vi "SYST_COMM_GPIB_RDEV_OPEN.vi"(0 "VISA IN":refnum<visa-resource-name>, 1 "Address":i32, 2 "Timeout":i32, 5 "error in":errorcluster, 7 "Bus":i32) -> (14 "VISA Out":refnum<visa-resource-name>, 19 "error out":errorcluster)   [LabVIEW 2018, in "PNA-X.lvlib"]
doc: "SYSTem:COMMunicate:GPIB:RDEVice:OPEN <bus>, <addr>, <timeout> \n(Read-Write) Initiates a GPIB pass-through session. First send this OPEN command, then send the \nOPEN query to read the session ID number. An existing GPIB pass-through session remains open \nafter an instrument preset. \nTo learn more about GPIB pass-through capability, see the example program. \nParameters \n<bus> Bus ID number. You can find the USB-GPIB adapter bus number by looking at \nthe dialog that appears when the USB-GPIB device is connected. Error 1073 \nindicates the bus or address number is incorrect. \n<addr> GPIB Address of the device to be controlled \n<timeout> The amount of time (in milliseconds) to wait for a response from the remote \ndevice after sending a command. A \"timeout\" error is displayed after this time \nhas passed without a response. \nExamples See an example program \nQuery Syntax SYSTem:COMMunicate:GPIB:RDEVice:OPEN? \nReturns the session identification number that is used when communicating \nwith this device. \nReturn Type Numeric \nDefault Not Applicable"
uses:
  PNA-X.lvlib
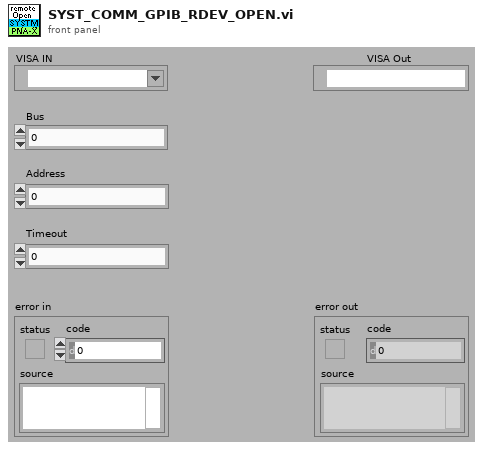
[diagram p1: front panel]
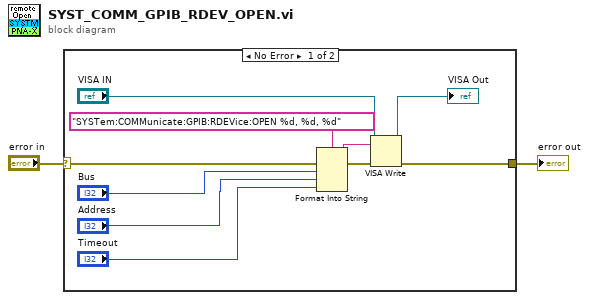
[diagram p0: block diagram]
diagram:
  n1 = case shown="No Error" "error in" {
    selector: "error in" -> [w12 w13]
    tunnel: [w7 w13] -> w1
    frame No Error {
      n2 = Format Into String(format string="SYSTem:COMMunicate:GPIB:RDEVice:OPEN %d, %d, %d" ("Cmdline"), error in=w12, "Bus", "Address", "Timeout") -> (resulting string=w10:string, error out=w11:errorcluster)  [unwired: 1 in]
      n3 = VISA Write(VISA resource name="VISA IN", write buffer=w10, error in (no error)=w11) -> (VISA resource name out=→"VISA Out":refnum<visa-resource-name>, error out=w7:errorcluster)  [unwired: 1 out]
    }
    frame Error {
    }
  }
  "error out" <- w1
